vi "new_pigeon_status_period.vi"(8 "error in (no error)":errorcluster, 11 "PigeonIMUDevRef In":T1={"DeviceStatus"={"status"=FALSE, "code"=0, "source"=""}, "Device Number"=0, "Type"=352321536, "Device ID"=0, "Handle"=0, "UsageFrame"=0, "Library Path"=path ""} {"Type" items=["CAN"=352321536, "TalonSRX"=33554432]}) -> (0 "error out":errorcluster, 3 "PigeonIMUDevRef Out":T1={"DeviceStatus"={"status"=FALSE, "code"=0, "source"=""}, "Device Number"=0, "Type"=352321536, "Device ID"=0, "Handle"=0, "UsageFrame"=0, "Library Path"=path ""} {"Type" items=["CAN"=352321536, "TalonSRX"=33554432]})   [LabVIEW 2020]
uses:
  <vilib>/Rock Robotics/WPI/ThirdParty/Phoenix-LabVIEW/Pigeon IMU/CTRE_PigeonIMU_DeviceRef.ctl
  <vilib>/Rock Robotics/WPI/ThirdParty/Phoenix-LabVIEW/Pigeon IMU/CTRE_PigeonIMU_ConnectionType.ctl
  <vilib>/Rock Robotics/WPI/ThirdParty/Phoenix-LabVIEW/Pigeon IMU/CTRE_PigeonIMU_StatusFrameRate.ctl
  <vilib>/ErrorRing/Error Ring.xnode
panel:
  in  "Tries":i32=3
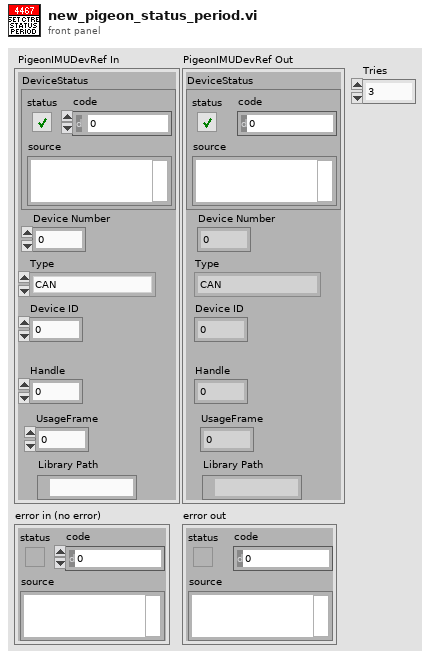
[diagram p1: front panel]
types:
  T1 = typedef "CTRE_PigeonIMU_DeviceRef.ctl" = cluster{"DeviceStatus":errorcluster, "Device Number":u8, "Type":T2, "Device ID":u32, "Handle":u64, "UsageFrame":u32, "Library Path":path}
  T2 = typedef "CTRE_PigeonIMU_ConnectionType.ctl" = u32
  T3 = typedef "CTRE_PigeonIMU_StatusFrameRate.ctl" = u32
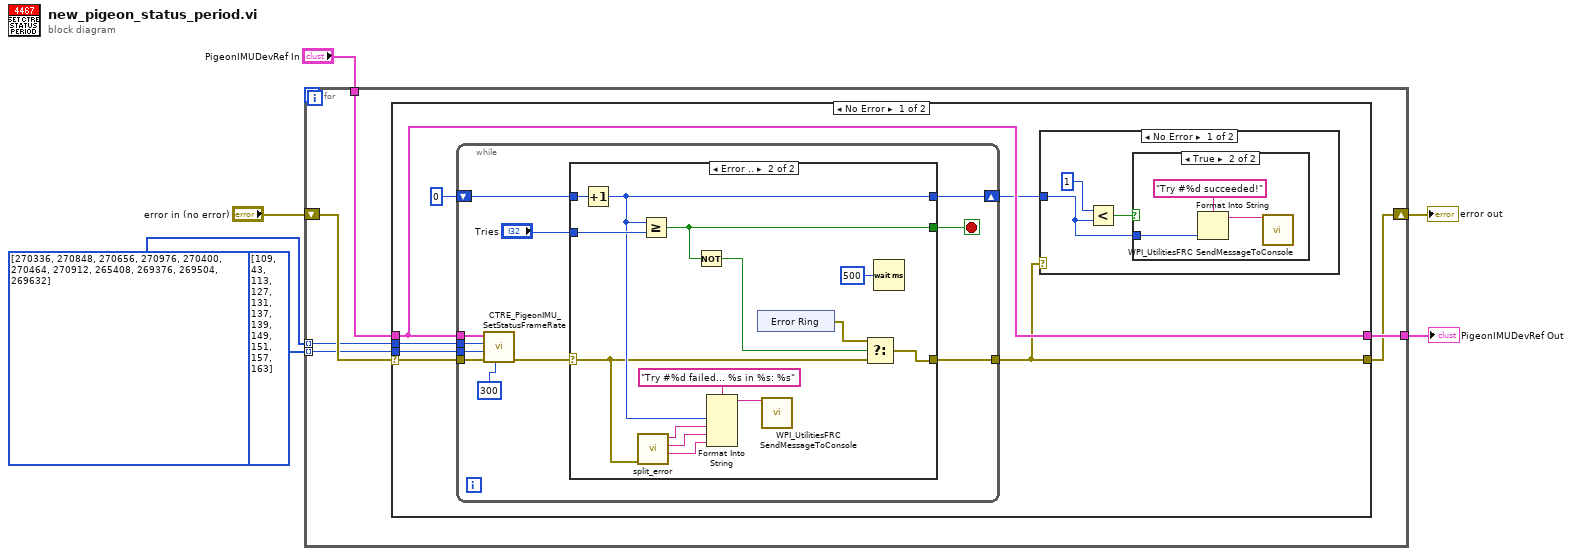
[diagram p0: block diagram]
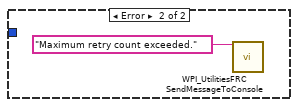
[diagram p3: hidden frame]
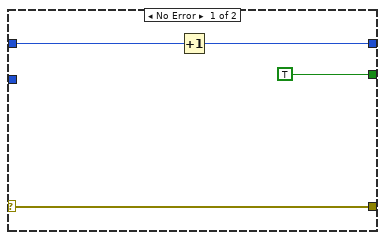
[diagram p4: hidden frame]
diagram:
  w3 = T3[] [270336, 270848, 270656, 270976, 270400, 270464, 270912, 265408, 269376, 269504, 269632] items=["CondStatus_1_General"=270336, "CondStatus_9_SixDeg_YPR"=270848, "CondStatus_6_SensorFusion"=270656, "CondStatus_11_GyroAccum"=270976, "CondStatus_2_GeneralCompass"=270400, "CondStatus_3_GeneralAccel"=270464, "CondStatus_10_SixDeg_Quat"=270912, "RawStatus_4_Mag"=265408, "BiasedStatus_2_Gyro"=269376, "BiasedStatus_4_Mag"=269504, "BiasedStatus_6_Accel"=269632] ("StatusFrame")
  n1 = for {
    tunnel: [w11] -> w6
    tunnel: "PigeonIMUDevRef In" -> [w12]
    tunnel: w3 -> [w7] mode=indexing
    tunnel: i16[] [109, 43, 113, 127, 131, 137, 139, 149, 151, 157, 163] -> [w8] mode=indexing
    shift-right: [w10] -> w5
    shift-left: "error in (no error)" -> [w9]
    n2 = case shown="No Error" w9 {
      selector: w9 -> [w15 w58]
      tunnel: [w13 w58] -> w10
      tunnel: [w16 w57] -> w11
      tunnel: w8 -> [w18 _]
      tunnel: w7 -> [w17 _]
      tunnel: w12 -> [w16 w57]
      frame No Error {
        n3 = while {
          shift-right: [w35] -> w14
          shift-left: 0 -> [w37]
          tunnel: [w34] -> w13
          tunnel: w15 -> [w33]
          tunnel: w18 -> [w27]
          tunnel: w17 -> [w28]
          tunnel: w16 -> [w32]
          stop <- w36 stop-if-true
          n4 = call <vilib>:"CTRE_PigeonIMU_SetStatusFrameRate.vi"("timeoutMs"=u32 300, "error in (no error)"=w33, "Period (ms)"=w27, "StatusFrame"=w28, "PigeonIMUDevRef"=w32) -> ("error out"=w31:errorcluster)  [unwired: 5 in, 1 out]
          n5 = case shown="Error .." w31 {
            selector: w31 -> [w39 w42]
            tunnel: w37 -> [w41 w55]
            tunnel: "Tries" -> [_ w54]
            tunnel: [TRUE w50] -> w36
            tunnel: [w38 w45] -> w35
            tunnel: [w39 w52] -> w34
            frame No Error {
              n6 = Increment(x=w41) -> (x+1=w38:i32)
            }
            frame Error {
              n7 = Increment(x=w55) -> (x+1=w45:i32)
              n8 = call "split_error.vi"("error in (no error)"=w42) -> ("callStack"=w46:string, "Location"=w47:string, "Details"=w48:string)  [unwired: 8 in]
              n9 = Greater Or Equal?(x=w45, y=w54) -> (x >= y?=w50:bool)
              n10 = Not(x=w50) -> (.not. x?=w43:bool)
              n11 = Format Into String(format string="Try #%d failed... %s in %s: %s", w45, w48, w47, w46) -> (resulting string=w44:string)  [unwired: 2 in, 1 out]
              n12 = xnode "Error Ring"() -> ("error out"=w51:errorcluster)
              n13 = call <vilib>:"WPI_UtilitiesFRC SendMessageToConsole.vi"("Message"=w44) -> ()  [unwired: 14 in, 1 out]
              n14 = Select(t=w51, s=w43, f=w42) -> (s? t:f=w52:errorcluster)
              n15 = Wait (ms)(milliseconds to wait=u32 500) -> ()  [unwired: 1 out]
            }
          }
        }
        n16 = case shown="No Error" w13 {
          tunnel: w14 -> [w21 _]
          frame No Error {
            n17 = Less?(x=1 ("y"), y=w21) -> (x < y?=w20:bool)
            n18 = case shown="True" w20 {
              tunnel: w21 -> [_ w24]
              frame False {
              }
              frame True {
                n19 = Format Into String(format string="Try #%d succeeded!", w24) -> (resulting string=w23:string)  [unwired: 2 in, 1 out]
                n20 = call <vilib>:"WPI_UtilitiesFRC SendMessageToConsole.vi"("Message"=w23) -> ()  [unwired: 14 in, 1 out]
              }
            }
          }
          frame Error {
            n21 = call <vilib>:"WPI_UtilitiesFRC SendMessageToConsole.vi"("Message"="Maximum retry count exceeded." ("format string")) -> ()  [unwired: 14 in, 1 out]
          }
        }
      }
      frame Error {
      }
    }
  }
  "error out" <- w5
  "PigeonIMUDevRef Out" <- w6
